vi "Prod - Rx.vi"(8 "Error In":errorcluster, 11 "Session Data In":T2={"MIDI-Messages"=[], "Rx-Data"=[], "Tx-Data"=[], "Session States"=enum."Wait to begin", "Tx Index"=0, "Communication Settings"={"Tx Protocol"=enum."Not Active", "Rx Protocol"=enum."Serial", "Serial"={"Tx Port"="", "Rx Port"="", "Baud rate"=8, "Parity"=enum."Space", "Data bits"=0, "Stop bits"=0, "Flow control"=enum."None", "Tx Resource"="", "Rx Resource"=""}, "MIDI Device"={"Input uDevice ID"=0, "Output uDevice ID"=0, "hmidiout Handle"=0, "hmidiin Handle"=0}, "Bluetooth"={"Dummy"=""}, "USB"={"Dummy"=""}}, "Timout-Time[ms]"=0, "Payload"=variant, "Queue_Session"=refnum, "To_GUI-Session"=refnum, "No More\nData"=FALSE, "Queue_Consumer"=refnum, "MIDI-Messages Log"=[], "Console log"=""}) -> (0 "Error Out":errorcluster, 3 "Session Data Out":T2={"MIDI-Messages"=[], "Rx-Data"=[], "Tx-Data"=[], "Session States"=enum."Wait to begin", "Tx Index"=0, "Communication Settings"={"Tx Protocol"=enum."Not Active", "Rx Protocol"=enum."Serial", "Serial"={"Tx Port"="", "Rx Port"="", "Baud rate"=8, "Parity"=enum."Space", "Data bits"=0, "Stop bits"=0, "Flow control"=enum."None", "Tx Resource"="", "Rx Resource"=""}, "MIDI Device"={"Input uDevice ID"=0, "Output uDevice ID"=0, "hmidiout Handle"=0, "hmidiin Handle"=0}, "Bluetooth"={"Dummy"=""}, "USB"={"Dummy"=""}}, "Timout-Time[ms]"=0, "Payload"=variant, "Queue_Session"=refnum, "To_GUI-Session"=refnum, "No More\nData"=FALSE, "Queue_Consumer"=refnum, "MIDI-Messages Log"=[], "Console log"=""})   [LabVIEW 2019]
doc: "Description of VI"
uses:
  Controls/Session_Data.ctl
  MIDI/Controls/MIDI-Message_Array.ctl
  MIDI/Controls/MIDI-Message_Cluster.ctl
  MIDI/Controls/Meta_Commands.ctl
  Controls/Session_State.ctl
  Common/Controls/Communication_Settings.ctl
  Common/Controls/Communication_Protocols.ctl
  Common/Controls/Application_Message.ctl
  Common/Controls/Application_State.ctl
  <vilib>/Utility/error.llb/DialogType.ctl
panel:
  in  "Control Tab":T1(tab)
  out "Error Message":string
  out "VI-filename":string
  out "VI Path":path
  out "Code Size":u32
  out "Revision Number":u32
  in  "Tool Bar:Visible":bool
  in  "Execution:Show Front Panel On Call":bool
  out "VI-Name":string
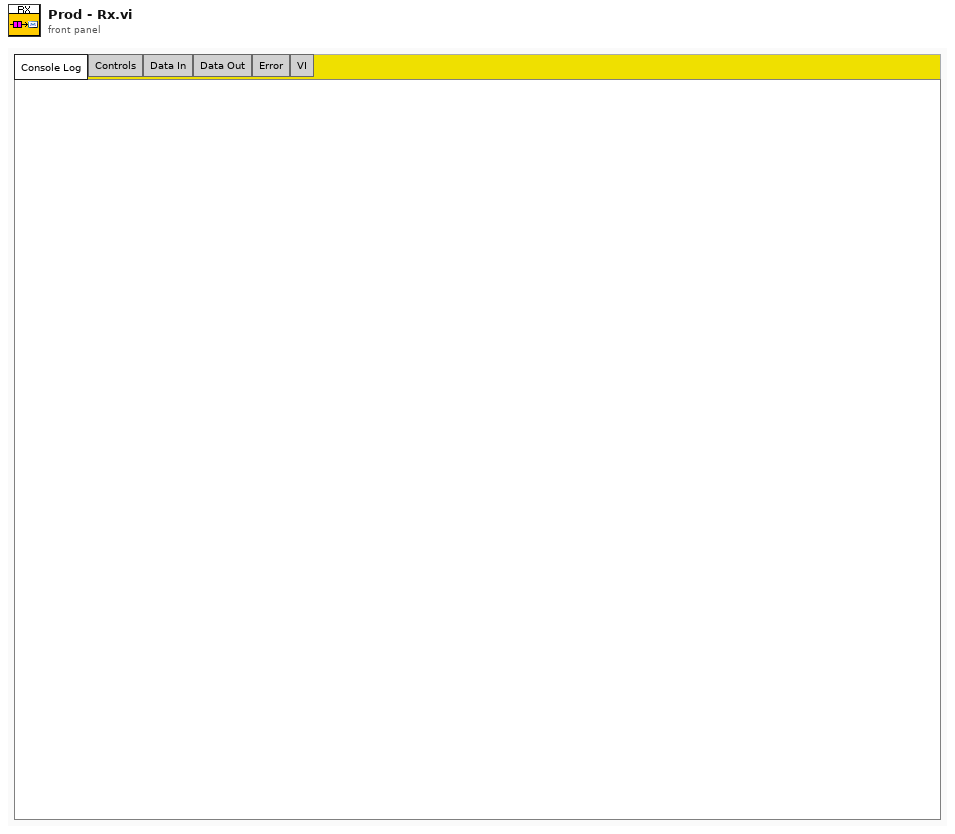
[diagram p1: front panel]
types:
  T1 = enum32{"Console Log", "Controls", "Data In", "Data Out", "Error", "VI"}
  T2 = typedef "Session_Data.ctl" = cluster{"MIDI-Messages":T3, "Rx-Data":i8[], "Tx-Data":i8[], "Session States":T6, "Tx Index":i32, "Communication Settings":T7, "Timout-Time[ms]":i32, "Payload":variant, "Queue_Session":refnum<queue>, "To_GUI-Session":refnum<user-event>, "No More\nData":bool, "Queue_Consumer":refnum<queue>, "MIDI-Messages Log":T3, "Console log":string}
  T3 = typedef "MIDI-Message_Array.ctl" = T4[]
  T4 = typedef "MIDI-Message_Cluster.ctl" = cluster{"Message Name":string, "Meta value":i32, "Datastring":string, "Datatype":T5}
  T5 = typedef "Meta_Commands.ctl" = enum16{"No Data", "Pause", "Loop", "Wait for Rx", "Delay", "Break", "MIDI"}
  T6 = typedef "Session_State.ctl" = enum16{"Wait to begin", "Active Session", "Pause", "Wait for Response", "Stop", "Restart", "Inspect", "Exit"}
  T7 = typedef "Communication_Settings.ctl" = cluster{"Tx Protocol":T8, "Rx Protocol":T8, "Serial":cluster{"Tx Port":refnum<visa-resource-name>, "Rx Port":refnum<visa-resource-name>, "Baud rate":i32, "Parity":enum16{"None", "Odd", "Even", "Mark", "Space"}, "Data bits":i32, "Stop bits":i32, "Flow control":enum16{"None", "XON/XOFF", "RTS/CTS", "XON/XOFF & RTS/CTS", "DTR/DSR", "XON/XOFF & DTR/DSR"}, "Tx Resource":refnum<visa-resource-name>, "Rx Resource":refnum<visa-resource-name>}, "MIDI Device":cluster{"Input uDevice ID":u32, "Output uDevice ID":u32, "hmidiout Handle":i32, "hmidiin Handle":i32}, "Bluetooth":cluster{"Dummy":string}, "USB":cluster{"Dummy":string}}
  T8 = typedef "Communication_Protocols.ctl" = enum16{"Serial", "Bluetooth", "USB-MIDI", "MIDI (Audio Device)", "Not Active"}
  T9 = typedef "DialogType.ctl" = u16
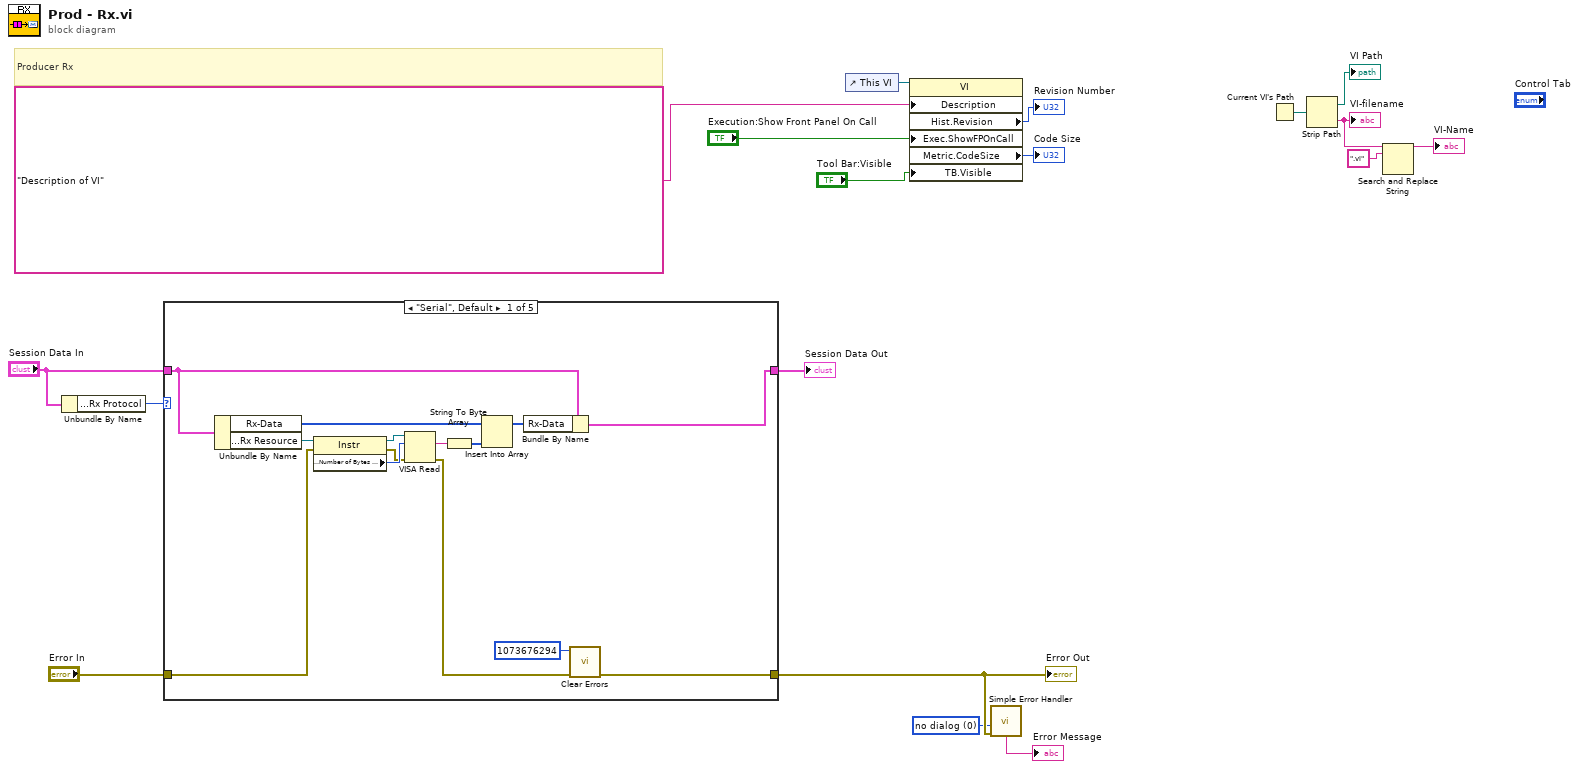
[diagram p0: block diagram]
diagram:
  w2 = T9 0 items=["no dialog", "OK message", "continue or stop message", "OK message + warnings", "continue/stop + warnings"] ("type of dialog (OK msg:1)")
  # "Producer Rx"
  n1 = Unbundle By Name("Session Data In") -> ("Communication Settings.Rx Protocol"=w7:T8)
  n2 = case shown="\"Serial\", Default" w7 {
    tunnel: "Session Data In" -> [w31 w34 w36 w37 w40]
    tunnel: "Error In" -> [w23 w33 w35 w38 w39]
    tunnel: [w19 w33 w35 w38 w39] -> w3
    tunnel: [w27 w34 w36 w37 w40] -> w4
    frame "Serial", Default {
      n3 = Unbundle By Name(w31) -> ("Rx-Data"=w30:i8[], "Communication Settings.Serial.Rx Resource"=w24:refnum<visa-resource-name>)
      n4 = property class="Instr"(reference=w24, error in=w23) -> (reference out=w22:refnum<visa-resource-name>, error out=w25:errorcluster, "Serial Settings:Number of Bytes at Serial Port"=w26:u32)
      n5 = VISA Read(VISA resource name=w22, byte count=w26, error in (no error)=w25) -> (read buffer=w32:string, error out=w21:errorcluster)  [unwired: 2 out]
      n6 = String To Byte Array(string=w32) -> (unsigned byte array=w29:u8[])
      n7 = Insert Into Array(array=w30, new element=w29) -> (w28:i8[])  [unwired: 1 in]
      n8 = Bundle By Name(cluster=w31, "Rx-Data"=w28) -> (w27:T2)
      n9 = call <vilib>:"Clear Errors.vi"("error in (no error)"=w21, "specific error code to clear (0: all)"=1073676294) -> ("error out"=w19:errorcluster)  [unwired: 4 in, 1 out]
    }
    frame "Bluetooth" {
    }
    frame "USB-MIDI" {
    }
    frame "MIDI (Audio Device)" {
      # "Is such a thing even possible?\n- Callback..."
    }
    frame "Not Active" {
    }
  }
  "Error Out" <- w3
  "Session Data Out" <- w4
  n10 = control-ref of="This VI"() -> (w12:refnum<vi>)
  n11 = property class="VI"(reference=w12, "Description"="Description of VI", "Exec.ShowFPOnCall"="Execution:Show Front Panel On Call", "TB.Visible"="Tool Bar:Visible") -> ("Hist.Revision"=→"Revision Number":u32, "Metric.CodeSize"=→"Code Size":u32)  [unwired: 1 in, 2 out]
  n12 = call <vilib>:"Simple Error Handler.vi"("type of dialog (OK msg:1)"=w2, "error in (no error)"=w3) -> ("message"=→"Error Message":string)  [unwired: 3 in, 4 out]
  n13 = Current VI's Path() -> (path=w18:path)
  n14 = Strip Path(path=w18) -> (stripped path=→"VI Path":path, name=w9:string)
  "VI-filename" <- w9
  n15 = Search and Replace String(input string=w9, search string=".vi") -> (result string=→"VI-Name":string)  [unwired: 6 in, 3 out]
